vi "Controller Operation Mode Management Loop.vi"(7 "Sync Objects":T1, 8 "error in (no error)":errorcluster, 11 "FOFB Configuration":T4={"FOFB Parameters"={"Network"={"FOFB Controller IP"="", "LNLS Control Network IP"="", "LNLS Control Network Power Supplies TCP Port"=0, "LNLS Control Network FOFB Configuration TCP Port"=0, "LNLS Control Network BPMs TCP Port"=0, "Data Server TCP Port"=0, "Monitoring Data TCP Port"=0, "Configuration GUI TCP Port"=0, "Storage Data TCP Port"=0, "Fast Command TCP Port"=0, "TCP Listening Timeout"=0, "Request Setpoints Rate"=0}, "Fast Acquisition"={"Acquisition Period"=0, "Data Buffer Size"=0, "Monitoring Period"=0}, "Response Matrix Measurement"={"Step Amplitude"=0.0, "Time Between Steps"=0, "Step Duration"=0, "Number of Averages"=0}, "Correction Algorithm"={"Correction Period"=0, "Reference Orbit Path"=path "", "Response Matrix Path"=path "", "Correction Matrix Path"=path "", "PID Horizontal Gain"=0.0, "PID Vertical Gain"=0.0, "PID Horizontal Integral Time"=0.0, "PID Vertical Integral Time"=0.0, "PID Horizontal Derivative Time"=0.0, "PID Vertical Derivative Time"=0.0, "Beam Current FOFB Threshold"=0.0, "Decouple H-V"=FALSE, "Use Additional BPM LPF"=FALSE, "BPM LPF Cutoff"=0.0}, "Acquisition Network"=[], "Actuation Network"=[]}, "Number of Acquisition Chassis"=0, "Number of Actuation Chassis"=0, "Number of BPM Readings"=0, "BPM Reading Names"=[], "Selected BPM Readings"=[0, 1, 2, 3, 4, 5, 6, 7, 8, 9, 10, 11, 12, 13, 14, 15, 16, 17, 18, 19, 20, 21, 22, 23, 24, 25, 26, 27, 28, 29, 30, 31, 32, 33, 34, 35, 36, 37, 38, 39, 40, 41, 42, 43, 44, 45, 46, 47, 48, 49], "Number of Correctors"=0, "Corrector Names"=[], "Selected Correctors"=[0, 1, 2, 3, 4, 5, 6, 7, 8, 9, 10, 11, 12, 13, 14, 15, 16, 17, 18, 19, 20, 21, 22, 23, 24, 25, 26, 27, 28, 29, 30, 31, 32, 33, 34, 35, 36, 37, 38, 39, 40, 41, 42, 43, 44, 45, 46, 47, 48, 49], "Reference Orbit"=[], "Response Matrix"=[], "Correction Matrix"=[], "Acquisition Chassis Names"=[], "Actuation Chassis Names"=[], "Acquisition Variables"=[], "Actuation Variables"=[], "PS Matrix Mapping"=[], "Inverse PS Matrix Mapping"=[], "BPM Matrix Mapping"=[], "Inverse BPM Matrix Mapping"=[], "Response Matrix Beam Energy (MeV)"=0.0, "PID Parameters"=[], "BPM Planes"=[], "Corrector Planes"=[], "RMM Step Factor"=[]}) -> (0 "error out":errorcluster)   [LabVIEW 2011, in "Controller VIs.lvlib"]
uses:
  Controller VIs.lvlib
  Types Definitions/Type FOFB Configuration.ctl
  Types Definitions/Type FOFB Parameters.ctl
  Types Definitions/Type Network Configuration.ctl
  Types Definitions/Type FA Configuration.ctl
  Types Definitions/Type Response Matrix Measurement Configuration.ctl
  Types Definitions/Type Correction Algorithm Configuration.ctl
  Types Definitions/Type Acquisition Network Configuration.ctl
  Types Definitions/Type Actuation Network Configuration.ctl
  Types Definitions/Type PID Parameters.ctl
  Types Definitions/Type Synchronization Objects.ctl
  Types Definitions/Type Blocking Synchronization Objects.ctl
  Types Definitions/Type Monitoring Data.ctl
  Types Definitions/Type Operation Mode State.ctl
  Types Definitions/Type Diagnostics Data.ctl
  Types Definitions/Type CPU Loads Array.ctl
  Types Definitions/Type CPU Loads.ctl
  Types Definitions/Type Non-blocking Synchronization Objects.ctl
  Types Definitions/Type FOFB Variables.ctl
  Types Definitions/Type Actuation State.ctl
  <vilib>/Platform/TimedLoop/XDataNode/timing_clust.ctl
  <vilib>/Platform/TimedLoop/XDataNode/nitl_modes.ctl
  <vilib>/Platform/TimedLoop/XDataNode/wakeup.ctl
  Controller Global Variables/LNLS Control FOFB Configuration In.vi
  Controller Global Variables/LNLS Control FOFB Configuration Out.vi
  <vilib>/Platform/TimedLoop/XDataNode/XDataNode.xnode
  Type Definitions.lvlib
  <vilib>/Platform/TimedLoop/XDataNode/XDNodeRunTimeDep.lvlib
  Controller Global Variables.lvlib
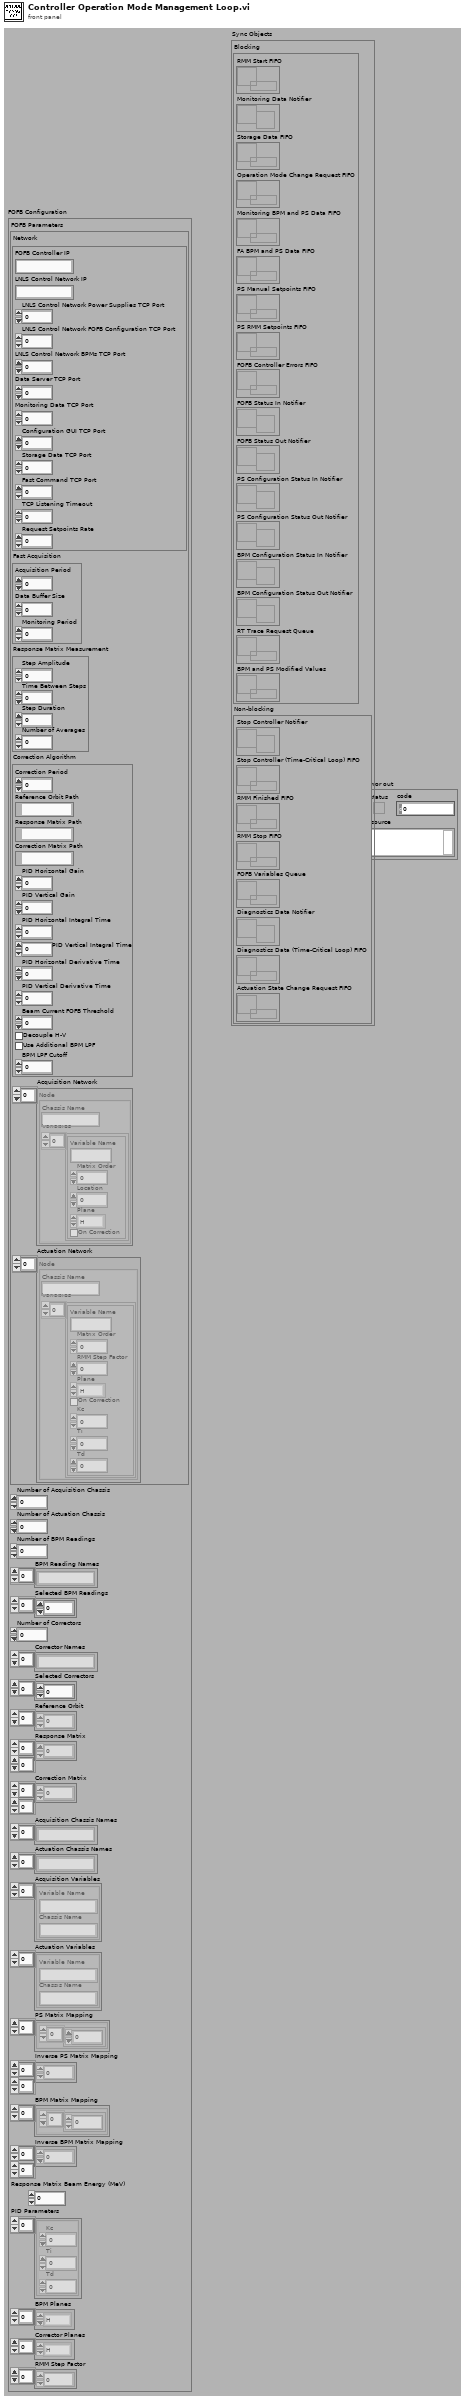
[diagram p1: front panel]
types:
  T1 = typedef "Type Definitions.lvlib/Type Synchronization Objects.ctl" = cluster{"Blocking":T2, "Non-blocking":T3}
  T2 = typedef "Type Definitions.lvlib/Type Blocking Synchronization Objects.ctl" = cluster{"RMM Start FIFO":refnum<k33>, "Monitoring Data Notifier":refnum<notifier>, "Storage Data FIFO":refnum<queue>, "Operation Mode Change Request FIFO":refnum<k33>, "Monitoring BPM and PS Data FIFO":refnum<k33>, "FA BPM and PS Data FIFO":refnum<k33>, "PS Manual Setpoints FIFO":refnum<k33>, "PS RMM Setpoints FIFO":refnum<k33>, "FOFB Controller Errors FIFO ":refnum<k33>, "FOFB Status In Notifier":refnum<notifier>, "FOFB Status Out Notifier":refnum<notifier>, "PS Configuration Status In Notifier":refnum<notifier>, "PS Configuration Status Out Notifier":refnum<notifier>, "BPM Configuration Status In Notifier":refnum<notifier>, "BPM Configuration Status Out Notifier":refnum<notifier>, "RT Trace Request Queue":refnum<queue>, "BPM and PS Modified Values":refnum<k33>}
  T3 = typedef "Type Definitions.lvlib/Type Non-blocking Synchronization Objects.ctl" = cluster{"Stop Controller Notifier":refnum<notifier>, "Stop Controller (Time-Critical Loop) FIFO":refnum<k33>, "RMM Finished FIFO":refnum<k33>, "RMM Stop FIFO":refnum<k33>, "FOFB Variables Queue":refnum<queue>, "Diagnostics Data Notifier":refnum<notifier>, "Diagnostics Data (Time-Critical Loop) FIFO":refnum<k33>, "Actuation State Change Request FIFO":refnum<k33>}
  T4 = typedef "Type Definitions.lvlib/Type FOFB Configuration.ctl" = cluster{"FOFB Parameters":T5, "Number of Acquisition Chassis":i32, "Number of Actuation Chassis":i32, "Number of BPM Readings":i32, "BPM Reading Names":string[], "Selected BPM Readings":u32[], "Number of Correctors":i32, "Corrector Names":string[], "Selected Correctors":u32[], "Reference Orbit":dbl[], "Response Matrix":dbl[][], "Correction Matrix":dbl[][], "Acquisition Chassis Names":string[], "Actuation Chassis Names":string[], "Acquisition Variables":cluster{"Variable Name":string, "Chassis Name":string}[], "Actuation Variables":cluster{"Variable Name":string, "Chassis Name":string}[], "PS Matrix Mapping":cluster{u32[]}[], "Inverse PS Matrix Mapping":u32[][], "BPM Matrix Mapping":cluster{u32[]}[], "Inverse BPM Matrix Mapping":u32[][], "Response Matrix Beam Energy (MeV)":dbl, "PID Parameters":T12[], "BPM Planes":enum8{"H", "V"}[], "Corrector Planes":enum8{"H", "V"}[], "RMM Step Factor":dbl[]}
  T5 = typedef "Type Definitions.lvlib/Type FOFB Parameters.ctl" = cluster{"Network":T6, "Fast Acquisition":T7, "Response Matrix Measurement":T8, "Correction Algorithm":T9, "Acquisition Network":T10, "Actuation Network":T11}
  T6 = typedef "Type Definitions.lvlib/Type Network Configuration.ctl" = cluster{"FOFB Controller IP":string, "LNLS Control Network IP":string, "LNLS Control Network Power Supplies TCP Port":u16, "LNLS Control Network FOFB Configuration TCP Port":u16, "LNLS Control Network BPMs TCP Port":u16, "Data Server TCP Port":u16, "Monitoring Data TCP Port":u16, "Configuration GUI TCP Port":u16, "Storage Data TCP Port":u16, "Fast Command TCP Port":u16, "TCP Listening Timeout":i32, "Request Setpoints Rate":u16}
  T7 = typedef "Type Definitions.lvlib/Type FA Configuration.ctl" = cluster{"Acquisition Period":u32, "Data Buffer Size":u32, "Monitoring Period":u32}
  T8 = typedef "Type Definitions.lvlib/Type Response Matrix Measurement Configuration.ctl" = cluster{"Step Amplitude":dbl, "Time Between Steps":u32, "Step Duration":u32, "Number of Averages":u32}
  T9 = typedef "Type Definitions.lvlib/Type Correction Algorithm Configuration.ctl" = cluster{"Correction Period":u32, "Reference Orbit Path":path, "Response Matrix Path":path, "Correction Matrix Path":path, "PID Horizontal Gain":dbl, "PID Vertical Gain":dbl, "PID Horizontal Integral Time":dbl, "PID Vertical Integral Time":dbl, "PID Horizontal Derivative Time":dbl, "PID Vertical Derivative Time":dbl, "Beam Current FOFB Threshold":dbl, "Decouple H-V":bool, "Use Additional BPM LPF":bool, "BPM LPF Cutoff":dbl}
  T10 = typedef "Type Definitions.lvlib/Type Acquisition Network Configuration.ctl" = cluster{"Chassis Name":string, "Variables":cluster{"Variable Name":string, "Matrix Order":u32, "Location":dbl, "Plane":enum8{"H", "V"}, "On Correction":bool}[]}[]
  T11 = typedef "Type Definitions.lvlib/Type Actuation Network Configuration.ctl" = cluster{"Chassis Name":string, "Variables":cluster{"Variable Name":string, "Matrix Order":u32, "RMM Step Factor":dbl, "Plane":enum8{"H", "V"}, "On Correction":bool, "Kc":dbl, "Ti":dbl, "Td":dbl}[]}[]
  T12 = typedef "Type Definitions.lvlib/Type PID Parameters.ctl" = cluster{"Kc":fxp<+/-,16,8>, "Ti":fxp<+/-,16,8>, "Td":fxp<+/-,16,8>}
  T13 = typedef "Type Definitions.lvlib/Type Operation Mode State.ctl" = enum8{"Idle Mode", "Manual Mode", "FOFB Mode", "RMM Mode"}
  T14 = typedef "XDNodeRunTimeDep.lvlib/timing_clust.ctl" = cluster{"Expected End [f-1]":u64, "Actual End [f-1]":u64, "Finished Late? [f-1]":bool, "Expected End [i-1]":u64, "Actual End [i-1]":u64, "Finished Late? [i-1]":bool, "Expected Start [i]":u64, "Actual Start [i]":u64, "Expected Start [f]":u64, "Actual Start [f]":u64, "Source Name":string, "Structure Name":string, "Period":i64, "Deadline":i64, "Offset":i64, "Start":i64, "Priority":i32, "Timeout":i32, "Mode":T15, "Wakeup Reason":T16, "Error":errorcluster, "Source Type":string, "Secondary Source Type":string, "Global End Time":u64, "Global Start Time":u64, "Frame Duration":u64, "Iteration Duration":u64, "Assigned CPU":i32, "I/O Scan Engine Mode":u32}
  T15 = typedef "XDNodeRunTimeDep.lvlib/nitl_modes.ctl" = enum32{"No Change", "Process missed periods, maintain original phase", "Discard missed periods, maintain original phase", "Process missed periods, ignore original phase", "Discard missed periods, ignore original phase"}
  T16 = typedef "XDNodeRunTimeDep.lvlib/wakeup.ctl" = enum32{"Normal", "Aborted", "Asynchronous wakeup", "Timing source error", "Timed loop error", "Timeout"}
  T17 = typedef "Type Definitions.lvlib/Type Actuation State.ctl" = enum8{"Only reading", "Manual", "FOFB Initialization", "FOFB", "FOFB Stopping", "RMM Initialization", "RMM", "RMM Stopping"}
  T18 = typedef "Type Definitions.lvlib/Type Control FOFB Configuration In.ctl" = cluster{"Status":u16, "Operation Mode":T13, "PID Horizontal Gain":sgl, "PID Vertical Gain":sgl, "PID Horizontal Integral Time":sgl, "PID Vertical Integral Time":sgl, "PID Horizontal Derivative Time":sgl, "PID Vertical Derivative Time":sgl, "Fast Command Enabled":bool}
  T19 = typedef "Type Definitions.lvlib/Type Control FOFB Configuration Out.ctl" = cluster{"Status":u16, "Operation Mode":T13, "PID Horizontal Gain":sgl, "PID Vertical Gain":sgl, "PID Horizontal Integral Time":sgl, "PID Vertical Integral Time":sgl, "PID Horizontal Derivative Time":sgl, "PID Vertical Derivative Time":sgl, "Fast Command Enabled":bool, "RMS Horizontal Distortion":dbl, "RMS Vertical Distortion":dbl, "Timestamp":dbl}
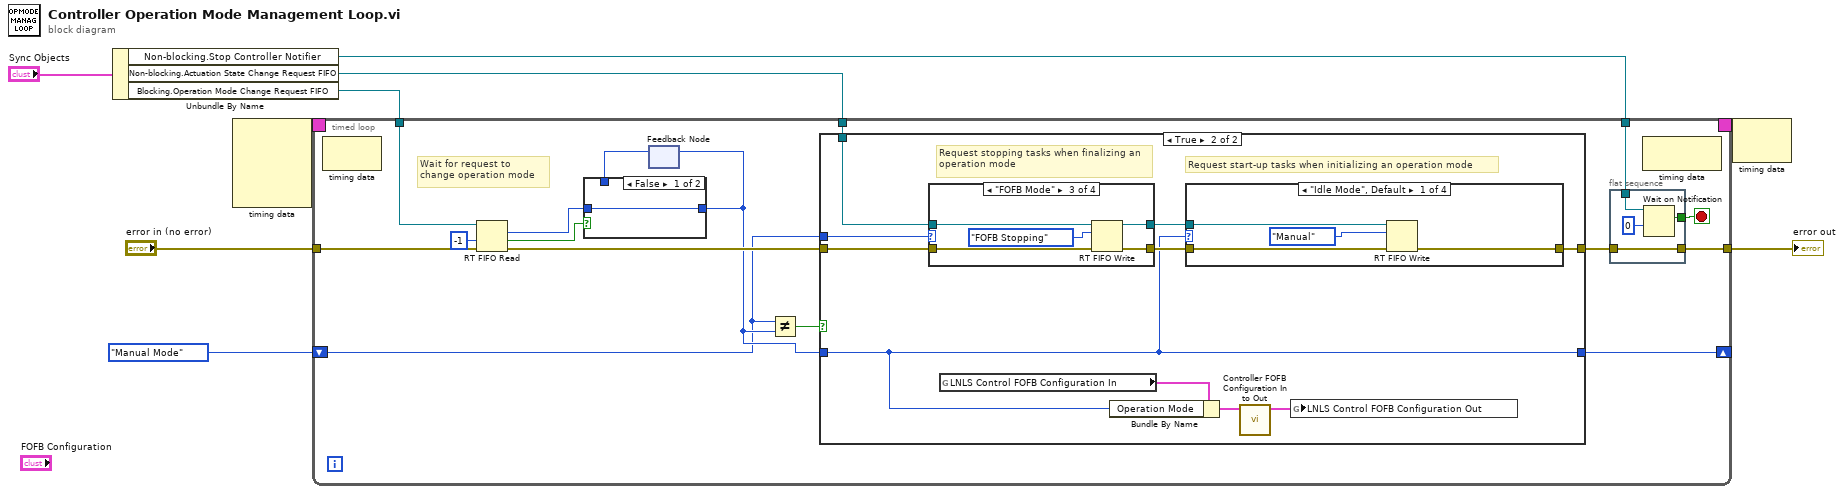
[diagram p0: block diagram]
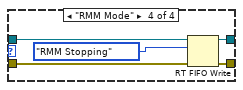
[diagram p6: hidden frame]
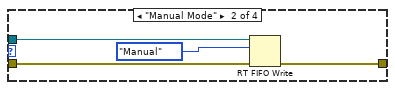
[diagram p7: hidden frame]
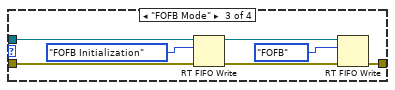
[diagram p8: hidden frame]
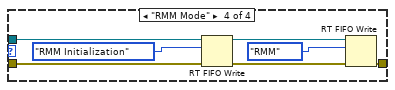
[diagram p9: hidden frame]
diagram:
  n1 = Unbundle By Name("Sync Objects") -> ("Non-blocking.Stop Controller Notifier"=w7:refnum<notifier>, "Non-blocking.Actuation State Change Request FIFO"=w3:refnum<k33>, "Blocking.Operation Mode Change Request FIFO"=w6:refnum<k33>)
  n2 = node-c288() -> (w2:T14)  [unwired: 4 in]
  n3 = timed-loop {
    tunnel: [w20] -> w9
    tunnel: "error in (no error)" -> [w22]
    tunnel: w7 -> [w24]
    shift-right: [w16] -> _
    shift-left: Type_Operation_Mode_State."Manual Mode" ("Operation Mode") -> [w10]
    tunnel: w6 -> [w23]
    tunnel: w3 -> [w21]
    timing: w2 -> [_]
    timing-out: [_] -> w1
    stop <- w25 stop-if-true
    # "Wait for request to \nchange operation mode"
    n4 = node-c288() -> ()  [unwired: 1 in, 1 out]
    n5 = RT FIFO Read(0:w23, 2:-1 ("timeout in ms (0)"), 3:w22) -> (9:w13:T13, 10:w12:bool, 11:w17:errorcluster)  [unwired: 1 in, 2 out]
    n6 = feedback #1() -> (w14:T13)  [unwired: 1 in]
    n7 = case shown="False" w12 {
      tunnel: [w26 w27] -> w15
      tunnel: w13 -> [w26 _]
      tunnel: w14 -> [_ w27]
      frame False {
      }
      frame True {
      }
    }
    n8 = feedback-in #1(w15) -> ()
    n9 = Not Equal?(x=w10, y=w15) -> (x != y?=w19:bool)
    n10 = case shown="True" w19 {
      tunnel: w15 -> [_ w34]
      tunnel: w21 -> [_ w41]
      tunnel: [w31 w38] -> w18
      tunnel: w17 -> [w31 w37]
      tunnel: [w30 w34] -> w16
      tunnel: w10 -> [w30 w36]
      frame False {
      }
      frame True {
        # "Request start-up tasks when initializing an operation mode"
        # "Request stopping tasks when finalizing an operation mode"
        n11 = case shown="\"FOFB Mode\"" w36 {
          tunnel: w41 -> [w42 w44 w50 w55]
          tunnel: w37 -> [w43 w45 w49 w54]
          tunnel: [w43 w45 w48 w53] -> w39
          tunnel: [w42 w44 w47 w52] -> w40
          frame "Idle Mode", Default {
          }
          frame "Manual Mode" {
          }
          frame "FOFB Mode" {
            n12 = RT FIFO Write(0:w50, 1:Type_Actuation_State."FOFB Stopping" ("element"), 3:w49) -> (8:w47:refnum<k33>, 11:w48:errorcluster)  [unwired: 2 in, 2 out]
          }
          frame "RMM Mode" {
            n13 = RT FIFO Write(0:w55, 1:Type_Actuation_State."RMM Stopping" ("element"), 3:w54) -> (8:w52:refnum<k33>, 11:w53:errorcluster)  [unwired: 2 in, 2 out]
          }
        }
        n14 = global read "LNLS Control FOFB Configuration In.vi" "LNLS Control FOFB Configuration In"() -> (w35:T18)
        n15 = Bundle By Name(cluster=w35, "Operation Mode"=w34) -> (w33:T18)
        n16 = case shown="\"Idle Mode\", Default" w34 {
          tunnel: w40 -> [w59 w62 w68 w77]
          tunnel: w39 -> [w58 w63 w67 w75]
          tunnel: [w57 w61 w66 w73] -> w38
          frame "Idle Mode", Default {
            n17 = RT FIFO Write(0:w59, 1:Type_Actuation_State."Manual" ("element"), 3:w58) -> (11:w57:errorcluster)  [unwired: 2 in, 3 out]
          }
          frame "Manual Mode" {
            n18 = RT FIFO Write(0:w62, 1:Type_Actuation_State."Manual" ("element"), 3:w63) -> (11:w61:errorcluster)  [unwired: 2 in, 3 out]
          }
          frame "FOFB Mode" {
            n19 = RT FIFO Write(0:w68, 1:Type_Actuation_State."FOFB Initialization" ("element"), 3:w67) -> (8:w70:refnum<k33>, 11:w69:errorcluster)  [unwired: 2 in, 2 out]
            n20 = RT FIFO Write(0:w70, 1:Type_Actuation_State."FOFB" ("element"), 3:w69) -> (11:w66:errorcluster)  [unwired: 2 in, 3 out]
          }
          frame "RMM Mode" {
            n21 = RT FIFO Write(0:w77, 1:Type_Actuation_State."RMM Initialization" ("element"), 3:w75) -> (8:w76:refnum<k33>, 11:w74:errorcluster)  [unwired: 2 in, 2 out]
            n22 = RT FIFO Write(0:w76, 1:Type_Actuation_State."RMM" ("element"), 3:w74) -> (11:w73:errorcluster)  [unwired: 2 in, 3 out]
          }
        }
        n23 = call "Controller FOFB Configuration In to Out.vi"("LNLS Control FOFB Configuration In"=w33) -> ("LNLS Control FOFB Configuration Out"=w32:T19)  [unwired: 10 in]
        n24 = global write "LNLS Control FOFB Configuration Out.vi" "LNLS Control FOFB Configuration Out"(w32) -> ()
      }
    }
    n25 = flat-sequence {
      tunnel: [w81] -> w25
      tunnel: w24 -> [w80]
      tunnel: [w78] -> w20
      tunnel: w18 -> [w78]
      frame #0 {
        n26 = Wait on Notification(notifier=w80, timeout in ms (-1)=0) -> (notification=w81:bool)  [unwired: 2 in, 3 out]
      }
    }
    n27 = node-c288() -> ()  [unwired: 1 in, 1 out]
  }
  "error out" <- w9
  n28 = node-c288(w1) -> ()  [unwired: 1 out]
